vi "MaxY.vi"() -> ()   [LabVIEW 2013]
panel:
  in  "Max Y in":u32=1 step=1
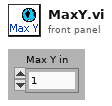
[diagram p1: front panel]
diagram:
